vi "Room_Create.vi"(0 "reference in":refnum<class "Room.lvclass">, 1 "Lights":refnum<class "Light.lvclass">[](array[class]), 2 "ACs":refnum<class "Air Conditioner.lvclass">[](array[class]), 3 "Securities":refnum<class "Security.lvclass">[](array[class]), 4 "MusicDevices":refnum<class "MusicDevice.lvclass">[](array[class]), 5 "Error In":errorcluster) -> (14 "reference out":refnum<class "Room.lvclass">, 19 "Error Out":errorcluster)   [LabVIEW 2024, in "Room.lvclass"]
uses:
  Room.lvclass
  Room.lvclass/Room.ctl
  Devices/Light_class/Light.lvclass
  Devices/Air Conditioner_class/Air Conditioner.lvclass
  Devices/Security_class/Security.lvclass
  Devices/MusicDevice_class/MusicDevice.lvclass
panel:
  # "Connector Pane"
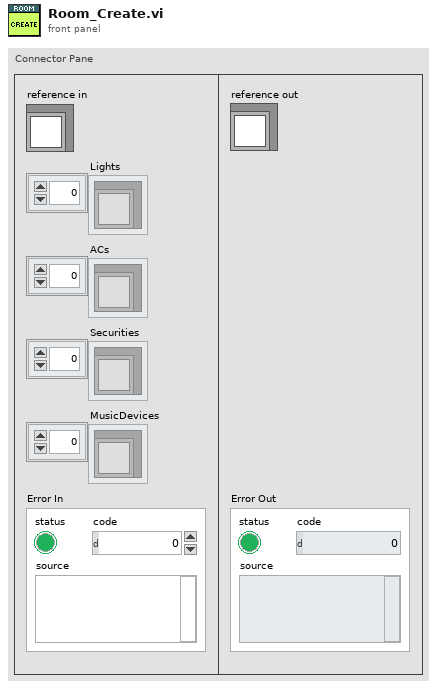
[diagram p1: front panel]
types:
  T1 = typedef "Room.lvclass/ObjectAttributes.ctl" = cluster{"Lights":refnum<class "Light.lvclass">[], "ACs":refnum<class "Air Conditioner.lvclass">[], "Securities":refnum<class "Security.lvclass">[], "MusicDevices":refnum<class "MusicDevice.lvclass">[]}
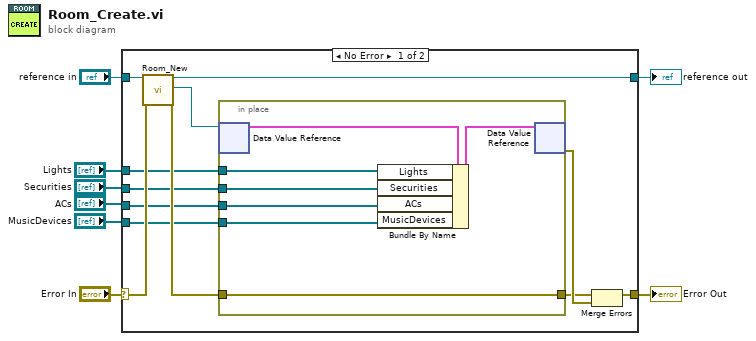
[diagram p0: block diagram]
diagram:
  n1 = case shown="No Error" "Error In" {
    selector: "Error In" -> [w19 w29]
    tunnel: [w16 w29] -> w7
    tunnel: "reference in" -> [w20 w28]
    tunnel: [w18 w28] -> w5
    tunnel: "MusicDevices" -> [w12 _]
    tunnel: "Securities" -> [w11 _]
    tunnel: "ACs" -> [w10 _]
    tunnel: "Lights" -> [w9 _]
    frame No Error {
      n2 = call "Room_New.vi"("reference in"=w20, "Error In"=w19) -> ("reference out"=w18:refnum<class "Room.lvclass">, "DVRRefOut"=w15:refnum<data-value>, "Error Out"=w14:errorcluster)  [unwired: 14 in, 1 out]
      n3 = in-place {
        in-place-border: w14 -> [w25]
        in-place-border: [w25] -> w13
        in-place-border: w12 -> [w24]
        in-place-border: w11 -> [w22]
        in-place-border: w10 -> [w21]
        in-place-border: w9 -> [w23]
        n4 = in-place-dvr #1(w15) -> (w26:T1)  [unwired: 1 out]
        n5 = Bundle By Name(cluster=w26, "Lights"=w23, "Securities"=w22, "ACs"=w21, "MusicDevices"=w24) -> (w27:T1)
        n6 = in-place-dvr #1(w27) -> (w17:errorcluster)  [unwired: 1 out]
      }
      n7 = Merge Errors(w13, w17) -> (w16:errorcluster)
    }
    frame Error {
      # "VI-TechBaseTemplate_Simple_6x8x6"
    }
  }
  "Error Out" <- w7
  "reference out" <- w5
